vi "03.1 deg2fah (subVI).vi"(1 "Degrees":dbl) -> (0 "Fahrenheit":dbl)   [LabVIEW 2019]
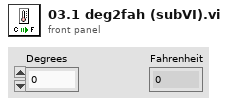
[diagram p1: front panel]
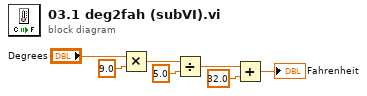
[diagram p0: block diagram]
diagram:
  n1 = Multiply(x="Degrees", y=9.0) -> (x*y=w3:dbl)
  n2 = Divide(x=w3, y=5.0) -> (x/y=w5:dbl)
  n3 = Add(x=w5, y=32.0) -> (x+y=→"Fahrenheit":dbl)
